vi "Manual Node Search.vi"(8 "error in (no error)":errorcluster, 10 "XPath Syntax":string, 11 "Node in":refnum<k20>) -> (0 "error out":errorcluster, 2 "Value":string, 3 "Node out":refnum<k20>)   [LabVIEW 2019, in "ParseSVG.lvclass"]
uses:
  ParseSVG.lvclass
  <vilib>/xml/Close Reference(NNMap).vi
  <vilib>/xml/Close Reference(Node).vi
  <resource>/objmgr/DOMUserDefRef.rc
  <vilib>/xml/NI_XML.lvlib
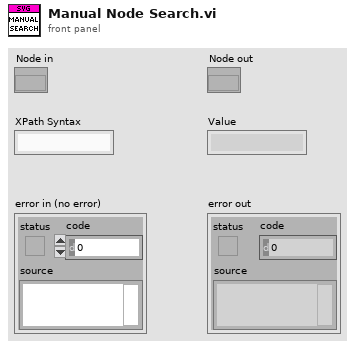
[diagram p1: front panel]
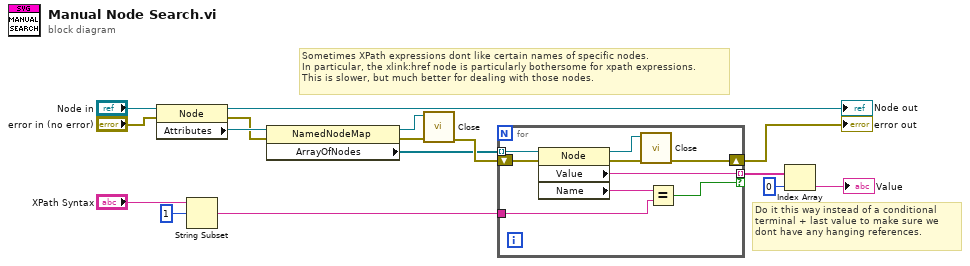
[diagram p0: block diagram]
diagram:
  # "Do it this way instead of a conditional terminal + last value to make sure we dont have any hanging references."
  # "Sometimes XPath expressions dont like certain names of specific nodes. \nIn particular, the xlink:href node is particularly bothersome for xpath expressions. \nThis is slower, but much better for dealing with those nodes."
  n1 = property class="Node"(reference="Node in", error in="error in (no error)") -> (reference out=→"Node out":refnum<k20>, error out=w8:errorcluster, "Attributes"=w11:refnum<k20>)
  n2 = String Subset(string="XPath Syntax", offset (0)=1) -> (substring=w12:string)  [unwired: 1 in]
  n3 = property class="NamedNodeMap"(reference=w11, error in=w8) -> (reference out=w6:refnum<k20>, error out=w10:errorcluster, "ArrayOfNodes"=w4:refnum<k20>[])
  n4 = call-poly <vilib>:"Close.vi"("error in (no error)"=w10, "named node map"=w6) -> ("error out"=w7:errorcluster)  [unwired: 7 in]
  n5 = for {
    tunnel: w4 -> [w25] mode=indexing
    tunnel: w12 -> [w18]
    tunnel: [w19] -> w2 mode=indexing if=w17
    shift-right: [w21] -> w9
    shift-left: w7 -> [w23]
    n6 = property class="Node"(reference=w25, error in=w23) -> (reference out=w20:refnum<k20>, error out=w22:errorcluster, "Value"=w19:string, "Name"=w24:string)
    n7 = call-poly <vilib>:"Close.vi"("error in (no error)"=w22, "node"=w20) -> ("error out"=w21:errorcluster)  [unwired: 7 in]
    n8 = Equal?(x=w24, y=w18) -> (x = y?=w17:bool)
  }
  "error out" <- w9
  n9 = Index Array(array=w2, index=0) -> (element=→"Value":string)
